vi "Read Timing Status.vi"(8 "error in (no error)":errorcluster, 11 "timing status pointer in":refnum<class "Timing Status.lvclass">) -> (0 "error out":errorcluster, 2 "timing status":T1 {"prev start time" format="%d us"; "cycle end time" format="%d us"; "cycle start time" format="%d us"; "tx end time" format="%d us"; "tx start time" format="%d us"; "rx end time" format="%d us"; "rx start time" format="%d us"}, 3 "timing status pointer out":refnum<class "Timing Status.lvclass">)   [LabVIEW 2017, in "DSF Core.lvlib" / "Timing Status.lvclass"]
uses:
  Timing Status.lvclass
  C:/Git/DSF/LabVIEW-Memory/Source/Classes/Pointer/Pointer.lvclass
  Timing Status Data.ctl
  LabVIEW-Memory/Source/Classes/Pointer/Pointer.lvclass
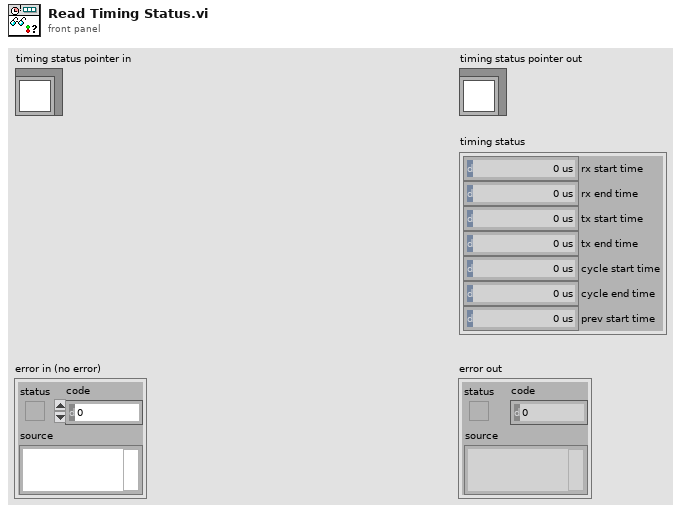
[diagram p1: front panel]
types:
  T1 = typedef "DSF Core.lvlib/Timing Status.lvclass/Timing Status Data.ctl" = cluster{"rx start time":u32, "rx end time":u32, "tx start time":u32, "tx end time":u32, "cycle start time":u32, "cycle end time":u32, "prev start time":u32}
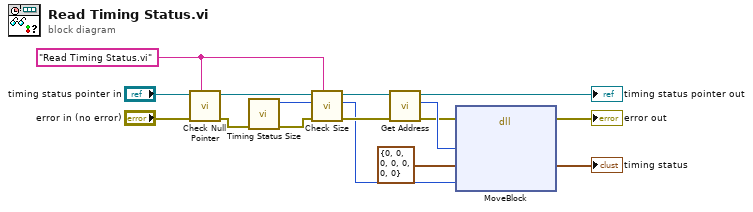
[diagram p0: block diagram]
diagram:
  w5 = "Read Timing Status.vi" ("source vi name")
  n1 = call "Check Null Pointer.vi"("source vi name"=w5, "error in (no error)"="error in (no error)", "Pointer in"="timing status pointer in") -> ("error out"=w7:errorcluster, "Pointer out"=w8:refnum<class "Timing Status.lvclass">)  [unwired: 7 in]
  n2 = call "Timing Status Size.vi"("error in (no error)"=w7) -> ("error out"=w10:errorcluster, "size"=w9:u64)  [unwired: 9 in]
  n3 = call "Check Size.vi"("source vi name"=w5, "error in (no error)"=w10, "required size"=w9, "Pointer in"=w8) -> ("error out"=w3:errorcluster, "required size out"=w1:u64, "Pointer out"=w2:refnum<class "Timing Status.lvclass">)  [unwired: 5 in]
  n4 = call "Get Address.vi"("Pointer in"=w2) -> ("address"=w15:u64, "Pointer out"=→"timing status pointer out":refnum<class "Timing Status.lvclass">)  [unwired: 9 in]
  n5 = dll-call lib="LabVIEW" fn="MoveBlock"(error in=w3, "src"=w15, "dst"=T1 {"rx start time"=0, "rx end time"=0, "tx start time"=0, "tx end time"=0, "cycle start time"=0, "cycle end time"=0, "prev start time"=0} ("Transfer Group status"), "size"=w1) -> (error out=→"error out":errorcluster, "dst"=→"timing status":T1)  [unwired: 5 in, 1 out]
